vi "OAT Easy Continuous Resampling.vi"   [LabVIEW 2017]
doc: "Resamples the even time-sampled <B>scaled signal [EU]</B> to an even angle-sampled signal. You can use this polymorphic VI to resample an analog tachometer signal or a digital tachometer signal. The data type you wire to the <B>analog tach signal</B> input determines the polymorphic instance to use."
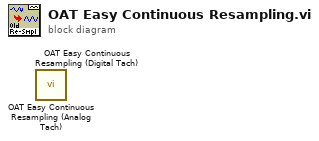
[diagram p0: block diagram]
diagram:
  n1 = call <vilib>:"OAT Easy Continuous Resampling (Analog Tach).vi"() -> ()  [unwired: 10 in, 6 out]
  n2 = call <vilib>:"OAT Easy Continuous Resampling (Digital Tach).vi"() -> ()  [unwired: 10 in, 6 out]
